vi "S. Distribute.vi"(6 "Variant in":variant, 7 "Shift Pressed?":bool, 8 "error in (no error)":errorcluster, 10 "QD Combo Box Ref":refnum<vi>, 11 "QD Launch VI Ref":refnum<vi>) -> (0 "error out":errorcluster, 4 "Variant out":variant)   [LabVIEW 2020]
doc: "Default Shortcut - [S]"
panel:
  in  "Undo Name":string="Quick Drop Keyboard Shortcut"
  # "Do not change the connector pane of this VI.\n\nSee the block diagram for directions on how to use this template."
  # "Specify the name of the Undo transaction"
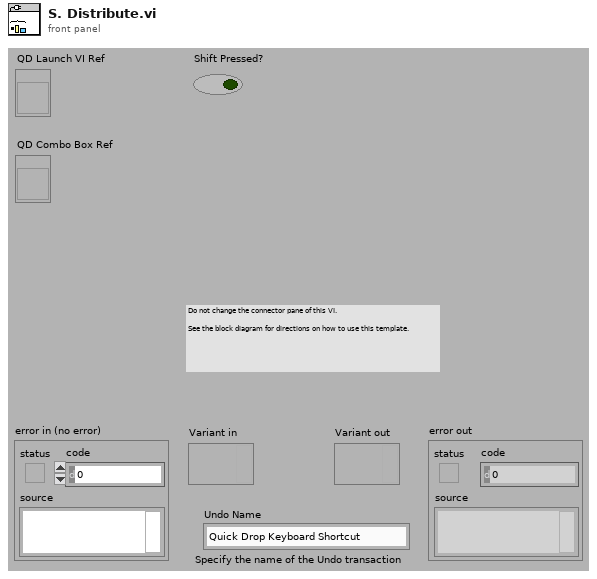
[diagram p1: front panel]
types:
  T1 = enum32{"Top Edges", "Vertical Centers", "Bottom Edges", "Vertical Gap", "Vertical Compress", "Left Edges", "Horizontal Centers", "Right Edges", "Horizontal Gap", "Horizontal Compress"}
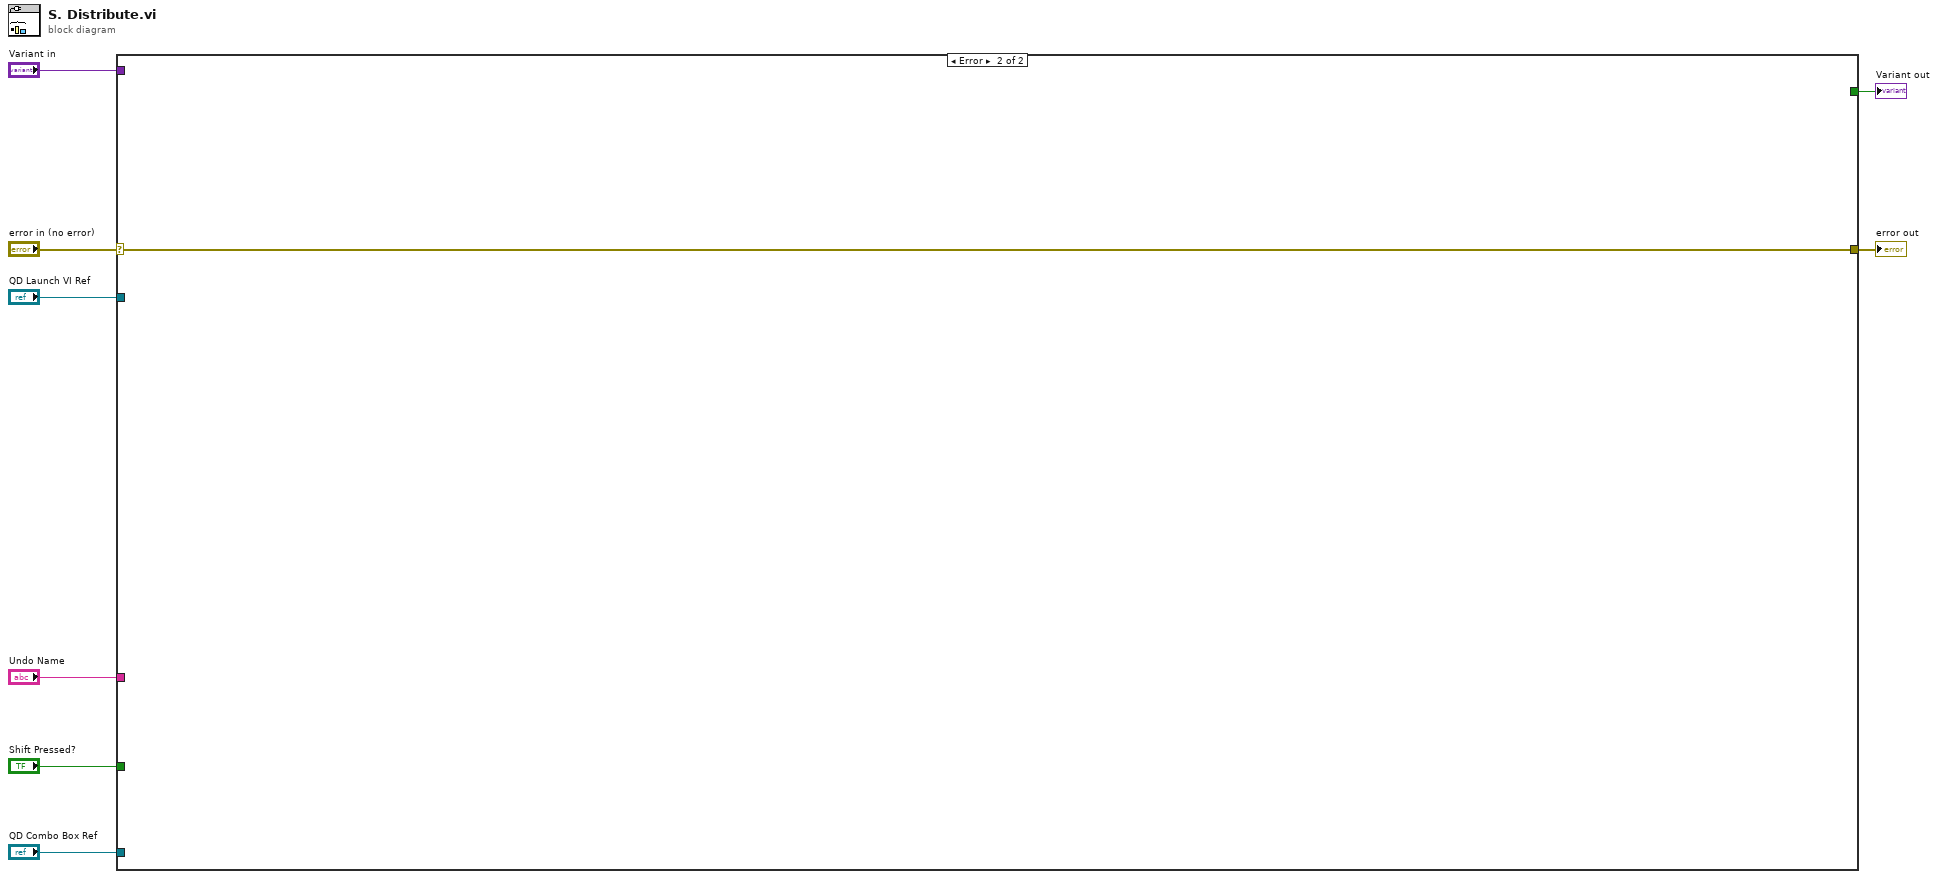
[diagram p0: block diagram]
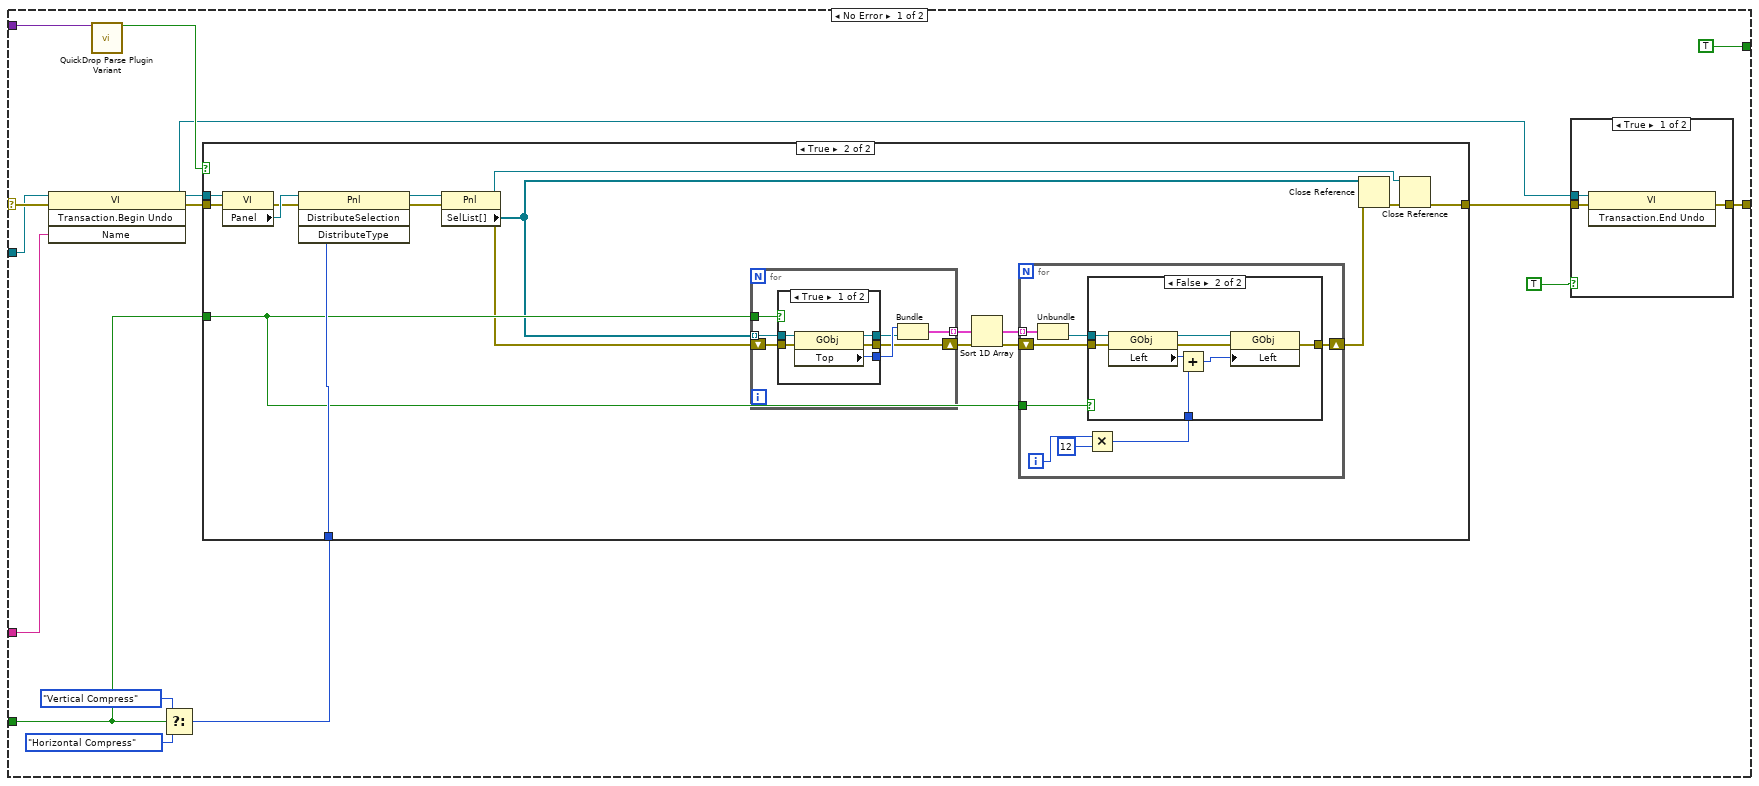
[diagram p2: hidden frame]
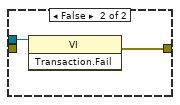
[diagram p3: hidden frame]
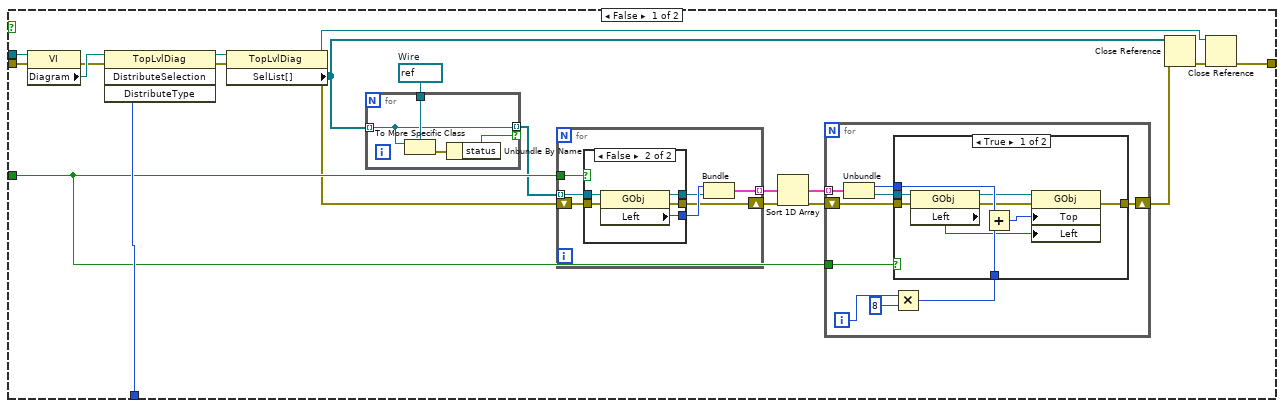
[diagram p4: hidden frame]
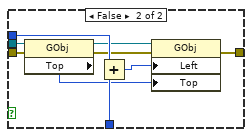
[diagram p5: hidden frame]
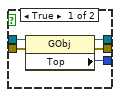
[diagram p6: hidden frame]
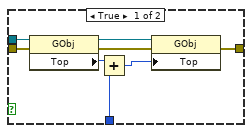
[diagram p7: hidden frame]
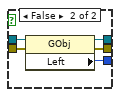
[diagram p8: hidden frame]
diagram:
  n1 = case shown="Error" "error in (no error)" {
    selector: "error in (no error)" -> [w22 w154]
    tunnel: [w16 w154] -> w7
    tunnel: "QD Launch VI Ref" -> [w21 _]
    tunnel: "Shift Pressed?" -> [w9 _]
    tunnel: "QD Combo Box Ref" -> [_ _]
    tunnel: "Variant in" -> [w23 _]
    tunnel: "Undo Name" -> [w20 _]
    tunnel: [TRUE _] -> w1
    frame No Error {
      n2 = invoke class="VI" method="Transaction.Begin Undo"(reference=w21, error in=w22, "Name"=w20) -> (reference out=w15:refnum<vi>, error out=w17:errorcluster)  [unwired: 1 in, 2 out]
      n3 = call <vilib>:"QuickDrop Parse Plugin Variant.vi"("QDKS Variant in"=w23) -> ("QD Launch VI Panel?"=w18:bool)  [unwired: 12 in, 2 out]
      n4 = Select(t=T1."Vertical Compress" ("DistributeType"), s=w9, f=T1."Horizontal Compress" ("DistributeType")) -> (s? t:f=w11:T1)
      n5 = case shown="True" w18 {
        tunnel: w17 -> [w47 w112]
        tunnel: w15 -> [w46 w111]
        tunnel: w11 -> [w42 w107]
        tunnel: [w41 w106] -> w10
        tunnel: w9 -> [w36 w101]
        frame False {
          w30 = refnum<vi> refnum  # Wire
          n6 = property class="VI"(reference=w46, error in=w47) -> (error out=w44:errorcluster, "Diagram"=w45:refnum<vi>)  [unwired: 1 out]
          n7 = invoke class="TopLvlDiag" method="DistributeSelection"(reference=w45, error in=w44, "DistributeType"=w42) -> (reference out=w40:refnum<vi>, error out=w43:errorcluster)  [unwired: 1 in, 2 out]
          n8 = property class="TopLvlDiag"(reference=w40, error in=w43) -> (reference out=w39:refnum<vi>, error out=w33:errorcluster, "SelList[]"=w31:refnum<vi>[])
          n9 = for {
            tunnel: w31 -> [w49] mode=indexing
            tunnel: w30 -> [w51]
            tunnel: [w49] -> w29 mode=indexing if=w48
            n10 = To More Specific Class(target class=w51, reference=w49) -> (error out=w50:errorcluster)  [unwired: 1 in, 1 out]
            n11 = Unbundle By Name(w50) -> ("status"=w48:bool)
          }
          n12 = for {
            tunnel: w29 -> [w85] mode=indexing
            tunnel: [w82] -> w38 mode=indexing
            tunnel: w36 -> [w81]
            shift-right: [w80] -> w32
            shift-left: w33 -> [w79]
            n13 = case shown="False" w81 {
              tunnel: w85 -> [w90 w95]
              tunnel: [w89 w94] -> w84
              tunnel: [w88 w93] -> w83
              tunnel: [w86 w92] -> w80
              tunnel: w79 -> [w87 w91]
              frame True {
                n14 = property class="GObj"(reference=w90, error in=w87) -> (reference out=w88:refnum<vi>, error out=w86:errorcluster, "Top"=w89:i32)
              }
              frame False {
                n15 = property class="GObj"(reference=w95, error in=w91) -> (reference out=w93:refnum<vi>, error out=w92:errorcluster, "Left"=w94:i32)
              }
            }
            n16 = Bundle("Left"=w84, w83) -> (w82:cluster{"Left":i32, refnum<vi>})  [unwired: 1 in]
          }
          n17 = Sort 1D Array(array=w38) -> (sorted array=w37:cluster{"Left":i32, refnum<vi>}[])
          n18 = for {
            tunnel: w37 -> [w60] mode=indexing
            tunnel: w36 -> [w59]
            shift-right: [w54] -> w34
            shift-left: w32 -> [w53]
            i -> [w57]
            n19 = Unbundle(w60) -> ("Left"=w52:i32, w58:refnum<vi>)
            n20 = Multiply(x=w57, y=8) -> (x*y=w56:i32)
            n21 = case shown="True" w59 {
              tunnel: w58 -> [w63 w72]
              tunnel: w56 -> [w68 w77]
              tunnel: [w67 w75] -> w54
              tunnel: w53 -> [w66 w76]
              tunnel: w52 -> [w65 w74]
              frame True {
                n22 = property class="GObj"(reference=w63, error in=w66) -> (reference out=w62:refnum<vi>, error out=w64:errorcluster, "Left"=w61:i32)
                n23 = Add(x=w65, y=w68) -> (x+y=w69:i32)
                n24 = property class="GObj"(reference=w62, error in=w64, "Top"=w69, "Left"=w61) -> (error out=w67:errorcluster)  [unwired: 1 out]
              }
              frame False {
                n25 = property class="GObj"(reference=w72, error in=w76) -> (reference out=w71:refnum<vi>, error out=w73:errorcluster, "Top"=w70:i32)
                n26 = Add(x=w74, y=w77) -> (x+y=w78:i32)
                n27 = property class="GObj"(reference=w71, error in=w73, "Left"=w78, "Top"=w70) -> (error out=w75:errorcluster)  [unwired: 1 out]
              }
            }
          }
          n28 = Close Reference(reference=w31, error in (no error)=w34) -> (error out=w35:errorcluster)
          n29 = Close Reference(reference=w39, error in (no error)=w35) -> (error out=w41:errorcluster)
        }
        frame True {
          n30 = property class="VI"(reference=w111, error in=w112) -> (error out=w109:errorcluster, "Panel"=w110:refnum<vi>)  [unwired: 1 out]
          n31 = invoke class="Pnl" method="DistributeSelection"(reference=w110, error in=w109, "DistributeType"=w107) -> (reference out=w105:refnum<vi>, error out=w108:errorcluster)  [unwired: 1 in, 2 out]
          n32 = property class="Pnl"(reference=w105, error in=w108) -> (reference out=w104:refnum<vi>, error out=w98:errorcluster, "SelList[]"=w96:refnum<vi>[])
          n33 = for {
            tunnel: w96 -> [w143] mode=indexing
            tunnel: [w140] -> w103 mode=indexing
            tunnel: w101 -> [w139]
            shift-right: [w138] -> w97
            shift-left: w98 -> [w137]
            n34 = case shown="True" w139 {
              tunnel: w143 -> [w148 w153]
              tunnel: [w147 w152] -> w142
              tunnel: [w146 w151] -> w141
              tunnel: [w144 w150] -> w138
              tunnel: w137 -> [w145 w149]
              frame True {
                n35 = property class="GObj"(reference=w148, error in=w145) -> (reference out=w146:refnum<vi>, error out=w144:errorcluster, "Top"=w147:i32)
              }
              frame False {
                n36 = property class="GObj"(reference=w153, error in=w149) -> (reference out=w151:refnum<vi>, error out=w150:errorcluster, "Left"=w152:i32)
              }
            }
            n37 = Bundle("Left"=w142, w141) -> (w140:cluster{"Left":i32, refnum<vi>})  [unwired: 1 in]
          }
          n38 = Sort 1D Array(array=w103) -> (sorted array=w102:cluster{"Left":i32, refnum<vi>}[])
          n39 = for {
            tunnel: w102 -> [w120] mode=indexing
            tunnel: w101 -> [w119]
            shift-right: [w114] -> w99
            shift-left: w97 -> [w113]
            i -> [w117]
            n40 = Unbundle(w120) -> (w118:refnum<vi>)  [unwired: 1 out]
            n41 = Multiply(x=w117, y=12) -> (x*y=w116:i32)
            n42 = case shown="False" w119 {
              tunnel: w118 -> [w128 w136]
              tunnel: w116 -> [w124 w132]
              tunnel: [w123 w130] -> w114
              tunnel: w113 -> [w121 w129]
              frame True {
                n43 = property class="GObj"(reference=w128, error in=w121) -> (reference out=w127:refnum<vi>, error out=w122:errorcluster, "Top"=w126:i32)
                n44 = Add(x=w126, y=w124) -> (x+y=w125:i32)
                n45 = property class="GObj"(reference=w127, error in=w122, "Top"=w125) -> (error out=w123:errorcluster)  [unwired: 1 out]
              }
              frame False {
                n46 = property class="GObj"(reference=w136, error in=w129) -> (reference out=w135:refnum<vi>, error out=w131:errorcluster, "Left"=w134:i32)
                n47 = Add(x=w134, y=w132) -> (x+y=w133:i32)
                n48 = property class="GObj"(reference=w135, error in=w131, "Left"=w133) -> (error out=w130:errorcluster)  [unwired: 1 out]
              }
            }
          }
          n49 = Close Reference(reference=w96, error in (no error)=w99) -> (error out=w100:errorcluster)
          n50 = Close Reference(reference=w104, error in (no error)=w100) -> (error out=w106:errorcluster)
        }
      }
      n51 = case shown="True" TRUE {
        tunnel: w15 -> [w25 w27]
        tunnel: [w26 w28] -> w16
        tunnel: w10 -> [w24 _]
        frame True {
          n52 = invoke class="VI" method="Transaction.End Undo"(reference=w25, error in=w24) -> (error out=w26:errorcluster)  [unwired: 1 in, 2 out]
        }
        frame False {
          n53 = invoke class="VI" method="Transaction.Fail"(reference=w27) -> (error out=w28:errorcluster)  [unwired: 2 in, 2 out]
        }
      }
    }
    frame Error {
    }
  }
  "error out" <- w7
  "Variant out" <- w1
